vi "Straight-Line Equation.vi"() -> ()   [LabVIEW 2020]
panel:
  out "y":dbl
  in  "x":dbl
  in  "Y-Intercept (b)":dbl
  in  "Slope (m)":dbl
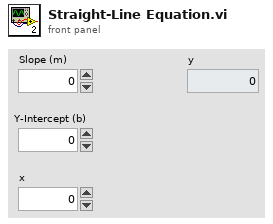
[diagram p1: front panel]
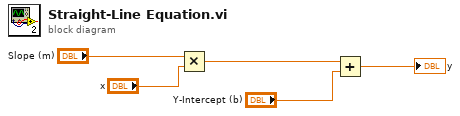
[diagram p0: block diagram]
diagram:
  n1 = Multiply(x="Slope (m)", y="x") -> (x*y=w5:dbl)
  n2 = Add(x=w5, y="Y-Intercept (b)") -> (x+y=→"y":dbl)
